vi "Kinesis - BPC303 - Two Axis Scan.vi"() -> ()   [LabVIEW 2012]
uses:
  U:/Software Training Plan/Software Training Day 2 - Thursday/Kinesis_with_LabVIEW_Examples_LV12 - v2/Thorlabs.MotionControl.Controls.dll
  Thorlabs.MotionControl.Controls.dll
  U:/Software Training Plan/Software Training Day 2 - Thursday/Kinesis_with_LabVIEW_Examples_LV12 - v2/Thorlabs.MotionControl.Benchtop.PiezoCLI.dll
  Thorlabs.MotionControl.Benchtop.PiezoCLI.dll
panel:
  in  "Wait Time (ms)":dbl=5000.0
  in  "Both Channels":i32
  in  "Scale":dbl=1.0
  in  "Num of Steps":i32=10
  in  "Channel B":i32=2
  out "Error":errorcluster
  in  "Channel A":i32=1
  in  "HWSerialNumA":string
  in  "BenchtopPiezoB":refnum<k24>(container)
  in  "BenchtopPiezoA":refnum<k24>(container)
  # "Notes:"
  # "- Ensure that the appropriate .DLLs are copied into your Project Folder. Check that the correct bit type are used depending on your version of LabVIEW\ni.e. 32-bit or 64-bit.\n\n\n\n\n\n\n\n\n\n\n\n\n\n\n- Open the example VI through the LabVIEW Project Explorer to correctly load the User Interface from Thorlabs.MotionControl.Controls.dll."
  # "Thorlabs Hardware: BPC303 Benchtop Piezo Controller\nhttps://www.thorlabs.com/newgrouppage9.cfm?objectgroup_id=1912&pn=BPC303#5457\n\nDescription: This VI will enable you to perform a 2D square raster scan on pre-selected channels on a BPC303 unit. This VI also includes the Error Handling cluster, able to print Error Messages & corresponding codes into this cluster.\n\nInstructions: \n1) Connect your BPC303 to your PC & power the device. For full device setup, the device product manual can be found on our website here. - https://www.thorlabs.com/thorproduct.cfm?partnumber=BPC303\n3) Enter the device serial number below.\n3) Edit the Scan Parameters: Step Size, Number of Steps, Scale (multiples of voltage steps) & Wait Time.\n4) To run the VI, click the run button in the LabVIEW toolbar.\n5) To end the VI, click 'END' to safely disconnect the device."
  # "Example Image of .NET Controller - VI opened via Project Explorer/ not opened via Project Explorer"
  # "VI Not Opened via Project Explorer"
  # "VI Opened via Project Explorer"
  # "- To explore the range of methods available, please visit the .NET API, included with your Kinesis software.\n\n- For tips on building your own VIs with Thorlabs Motion Control Hardware, please see our LabVIEW Guide here.\nhttps://www.thorlabs.com/newgrouppage9.cfm?objectgroup_id=10285"
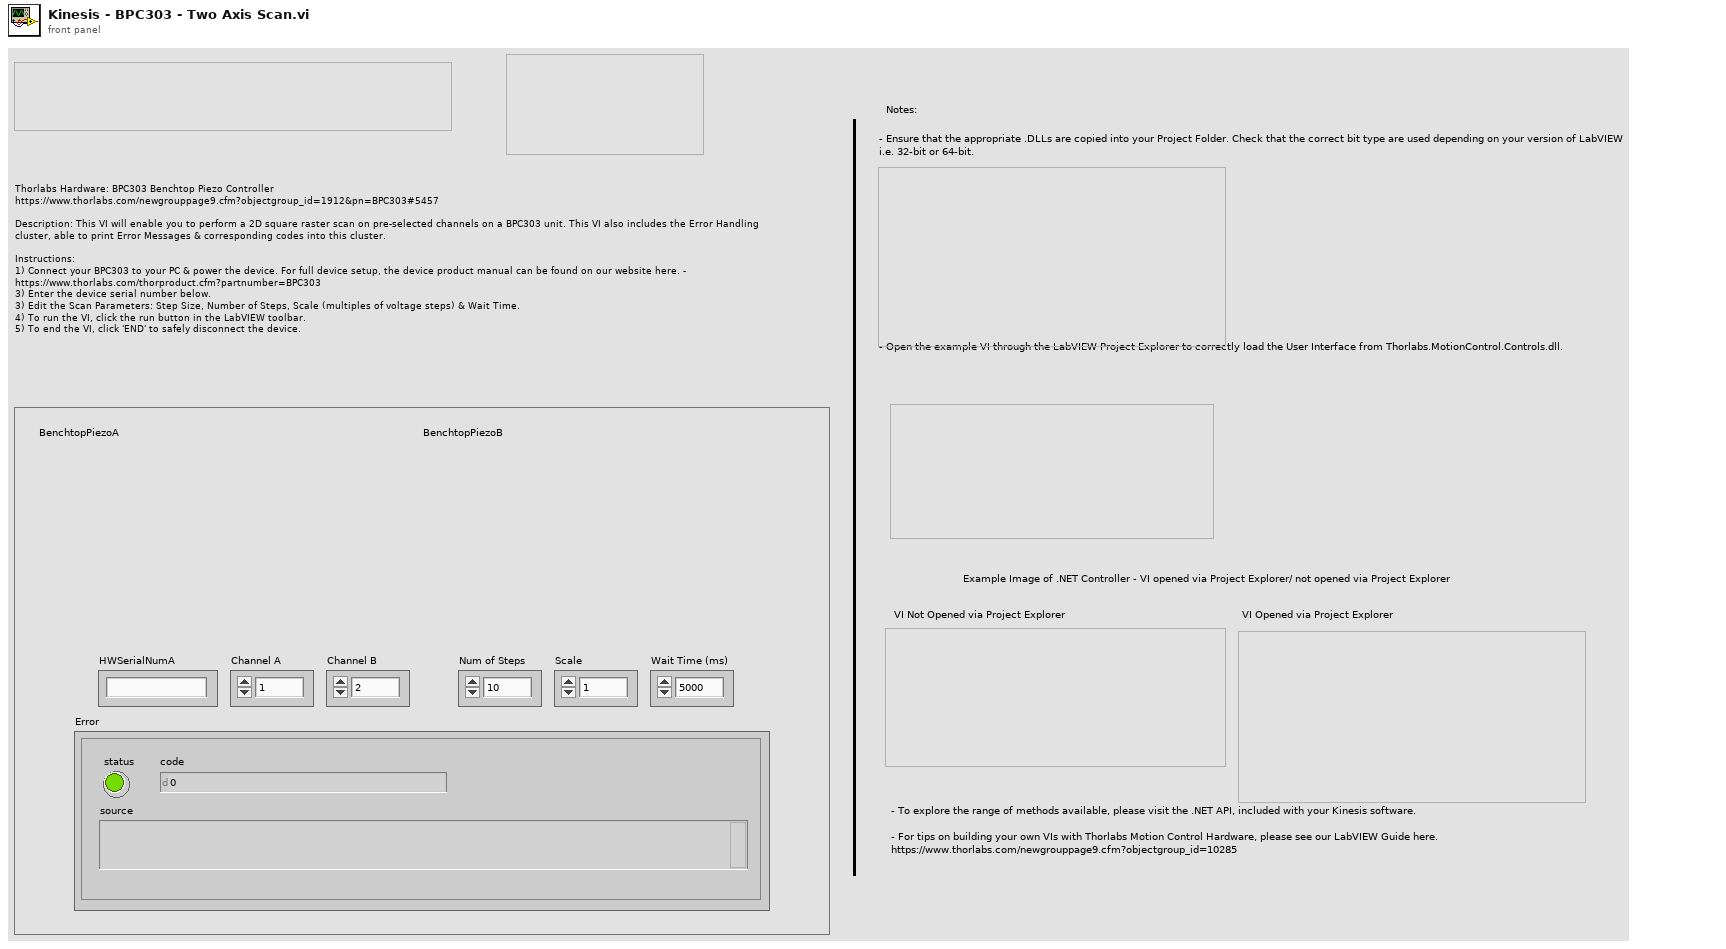
[diagram p1: front panel]
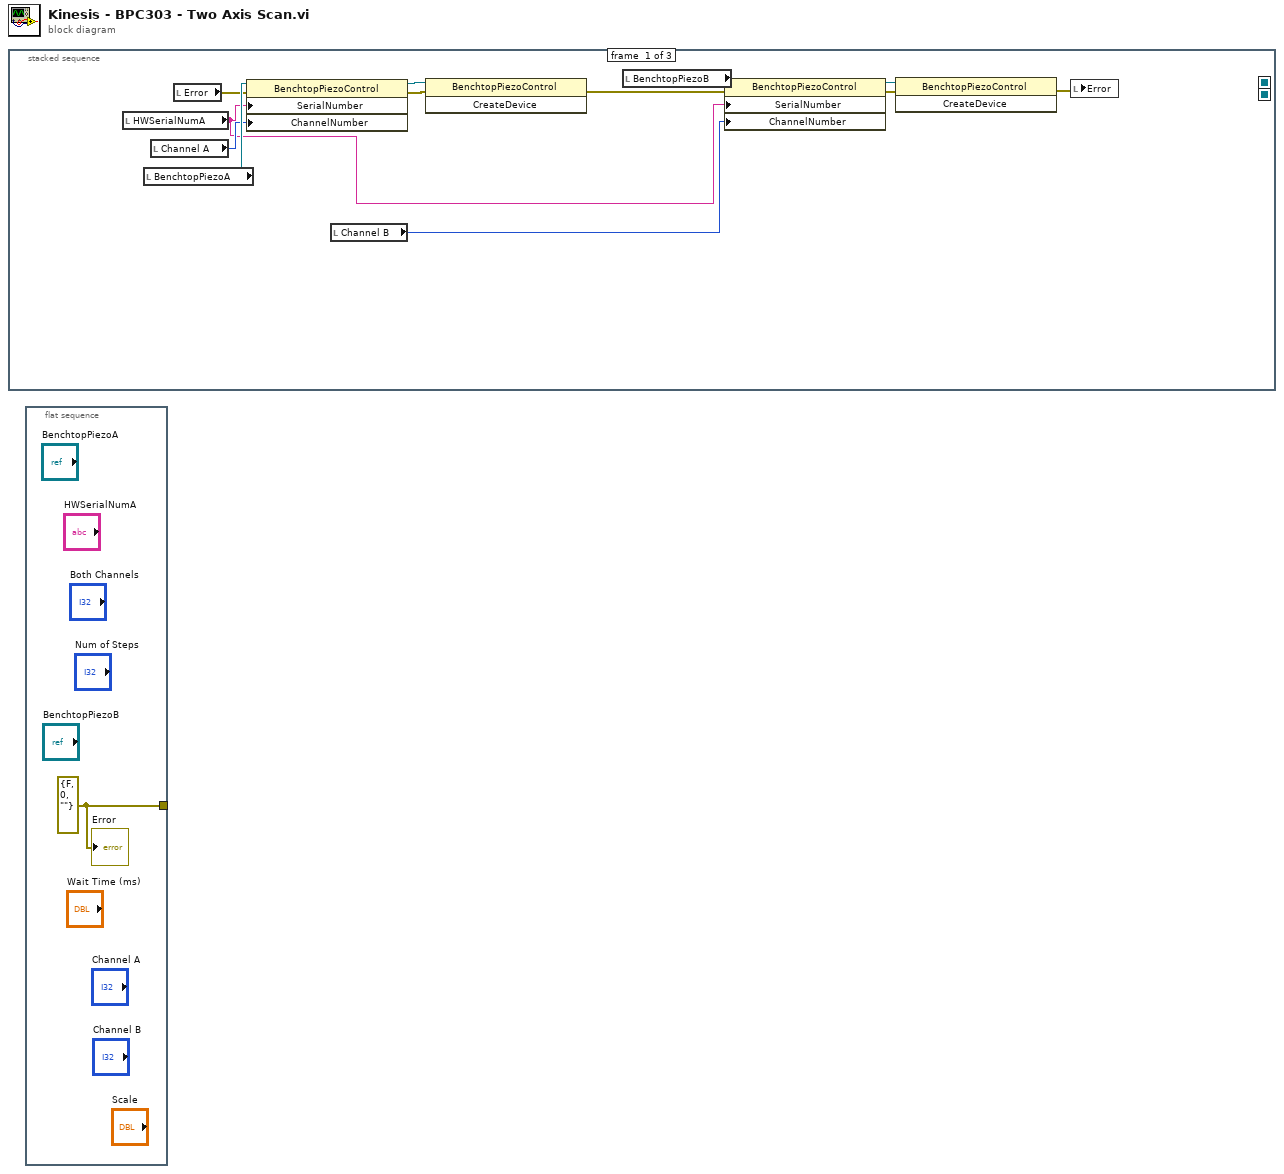
[diagram p0: block diagram]
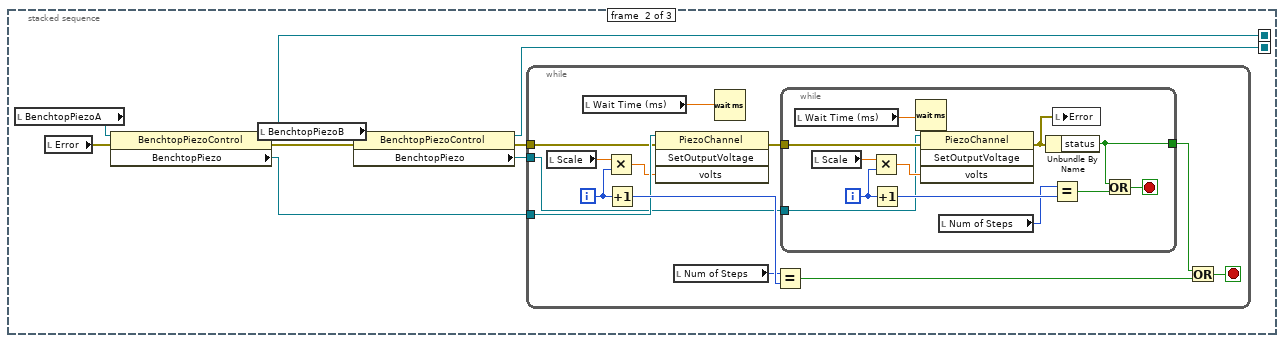
[diagram p2: hidden frame]
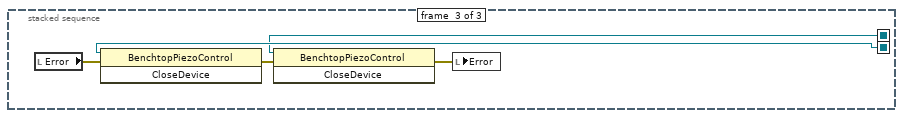
[diagram p3: hidden frame]
diagram:
  n1 = stacked-sequence {
    seq-local: [_ w19 _] -> [_ _ w51]
    seq-local: [_ w18 _] -> [_ _ w50]
    frame #0 {
      n2 = local read "HWSerialNumA"() -> (w7:string)
      n3 = local read "BenchtopPiezoA"() -> (w12:refnum<k24>)
      n4 = local read "Channel A"() -> (w8:i32)
      n5 = local read "Error"() -> (w10:errorcluster)
      n6 = property class="BenchtopPiezoControl"(reference=w12, error in=w10, "SerialNumber"=w7, "ChannelNumber"=w8) -> (reference out=w6:refnum<k24>, error out=w5:errorcluster)
      n7 = local read "Channel B"() -> (w9:i32)
      n8 = invoke class="BenchtopPiezoControl" method="CreateDevice"(reference=w6, error in=w5) -> (error out=w4:errorcluster)  [unwired: 1 in, 2 out]
      n9 = local read "BenchtopPiezoB"() -> (w11:refnum<k24>)
      n10 = property class="BenchtopPiezoControl"(reference=w11, error in=w4, "SerialNumber"=w7, "ChannelNumber"=w9) -> (reference out=w2:refnum<k24>, error out=w3:errorcluster)
      n11 = invoke class="BenchtopPiezoControl" method="CreateDevice"(reference=w2, error in=w3) -> (error out=w1:errorcluster)  [unwired: 1 in, 2 out]
      n12 = local write "Error"(w1) -> ()
    }
    frame #1 {
      n13 = local read "BenchtopPiezoA"() -> (w17:refnum<k24>)
      n14 = local read "Error"() -> (w16:errorcluster)
      n15 = property class="BenchtopPiezoControl"(reference=w17, error in=w16) -> (reference out=w18:refnum<k24>, error out=w14:errorcluster, "BenchtopPiezo"=w21:refnum<k24>)
      n16 = local read "BenchtopPiezoB"() -> (w15:refnum<k24>)
      n17 = property class="BenchtopPiezoControl"(reference=w15, error in=w14) -> (reference out=w19:refnum<k24>, error out=w13:errorcluster, "BenchtopPiezo"=w20:refnum<k24>)
      n18 = while {
        tunnel: w21 -> [w29]
        tunnel: w20 -> [w27]
        tunnel: w13 -> [w23]
        i -> [w34]
        stop <- w30 stop-if-true
        n19 = local read "Scale"() -> (w33:dbl)
        n20 = local read "Wait Time (ms)"() -> (w22:dbl)
        n21 = Multiply(x=w33, y=w34) -> (x*y=w28:dbl)
        n22 = Increment(x=w34) -> (x+1=w32:i32)
        n23 = invoke class="PiezoChannel" method="SetOutputVoltage"(reference=w29, error in=w23, "volts"=w28) -> (error out=w24:errorcluster)  [unwired: 1 in, 3 out]
        n24 = local read "Num of Steps"() -> (w31:i32)
        n25 = Wait (ms)(milliseconds to wait=w22) -> ()  [unwired: 1 out]
        n26 = Equal?(x=w31, y=w32) -> (x = y?=w26:bool)
        n27 = while {
          tunnel: w27 -> [w38]
          tunnel: w24 -> [w41]
          tunnel: [w36] -> w25
          i -> [w46]
          stop <- w39 stop-if-true
          n28 = local read "Wait Time (ms)"() -> (w35:dbl)
          n29 = local read "Scale"() -> (w45:dbl)
          n30 = Multiply(x=w45, y=w46) -> (x*y=w44:dbl)
          n31 = Increment(x=w46) -> (x+1=w43:i32)
          n32 = Wait (ms)(milliseconds to wait=w35) -> ()  [unwired: 1 out]
          n33 = invoke class="PiezoChannel" method="SetOutputVoltage"(reference=w38, error in=w41, "volts"=w44) -> (error out=w37:errorcluster)  [unwired: 1 in, 3 out]
          n34 = local read "Num of Steps"() -> (w42:i32)
          n35 = Unbundle By Name(w37) -> ("status"=w36:bool)
          n36 = Equal?(x=w42, y=w43) -> (x = y?=w40:bool)
          n37 = local write "Error"(w37) -> ()
          n38 = Or(x=w36, y=w40) -> (x .or. y?=w39:bool)
        }
        n39 = Or(x=w25, y=w26) -> (x .or. y?=w30:bool)
      }
    }
    frame #2 {
      n40 = local read "Error"() -> (w49:errorcluster)
      n41 = invoke class="BenchtopPiezoControl" method="CloseDevice"(reference=w51, error in=w49) -> (error out=w48:errorcluster)  [unwired: 1 in, 2 out]
      n42 = invoke class="BenchtopPiezoControl" method="CloseDevice"(reference=w50, error in=w48) -> (error out=w47:errorcluster)  [unwired: 1 in, 2 out]
      n43 = local write "Error"(w47) -> ()
    }
  }
  n44 = flat-sequence {
    tunnel: [w52] -> _
    frame #0 {
      w52 = errorcluster {"status"=FALSE, "code"=0, "source"=""} ("error in (no error)")
      "Error" <- w52
    }
  }
